vi "MLP_FS_ Target.vi"   [LabVIEW 2022 SP3]
uses:
  <vilib>/rvi/Emulation/niFpgaEmulationIsFPGAContextNoSignature.vi
  <vilib>/rvi/DataTransferAndStorage/Container/Common/niFpgaContainerGetUniqueNameForEmu.vi
  <vilib>/rvi/Memory/Memory_Emulation/niFpgaMemoryEmulationCacheClearOnFirstRun.vi
  <vilib>/rvi/Memory/Memory_Emulation/nirvimemoryEmulationManagerCache_MakeExclusive.vi
  <vilib>/rvi/Memory/Memory_Emulation/niFpgaMemoryEmulationValidateCache.vi
  <vilib>/rvi/Memory/Memory_Emulation/nirvimemoryEmulationManagerCache_InsertValue.vi
  <vilib>/Utility/error.llb/Clear Errors.vi
  <vilib>/rvi/Memory/Memory_Emulation/nirvimemoryEmulationManagerCache_ReleaseExclusive.vi
  <vilib>/rvi/Memory/Memory_Emulation/nirvimemoryEmulationManagerCache_GetValue.vi
  <vilib>/rvi/Memory/Memory_Emulation/nirvimemoryEmulationManagerCache_SetValue.vi
  <vilib>/rvi/Emulation/niFpgaProcessEmulError.vi
  <vilib>/rvi/Emulation/niFpgaSctlEmulationGetInTimedLoop.vi
  <vilib>/rvi/interface/RandomDataEmulation/niFpgaRandomDataHandleErrors.vi
  <vilib>/rvi/Memory/Memory_Emulation/nirvimemoryFastEmulation.vi
  <vilib>/rvi/Memory/Memory_Emulation/nirvimemoryEmulation.vi
  <vilib>/rvi/errors/nirviReportUnexpectedCaseInternalError (U32).vi
  <vilib>/rvi/DataTransferAndStorage/Container/XNode/niFpgaContainer.xnode
  <vilib>/rvi/DataTransferAndStorage/Register/Emulation/niFpgaRegisterEmulation.vi
  <vilib>/rvi/interface/RandomDataEmulation/nirviRandomDataFpgaReadWriteTemplate.vi
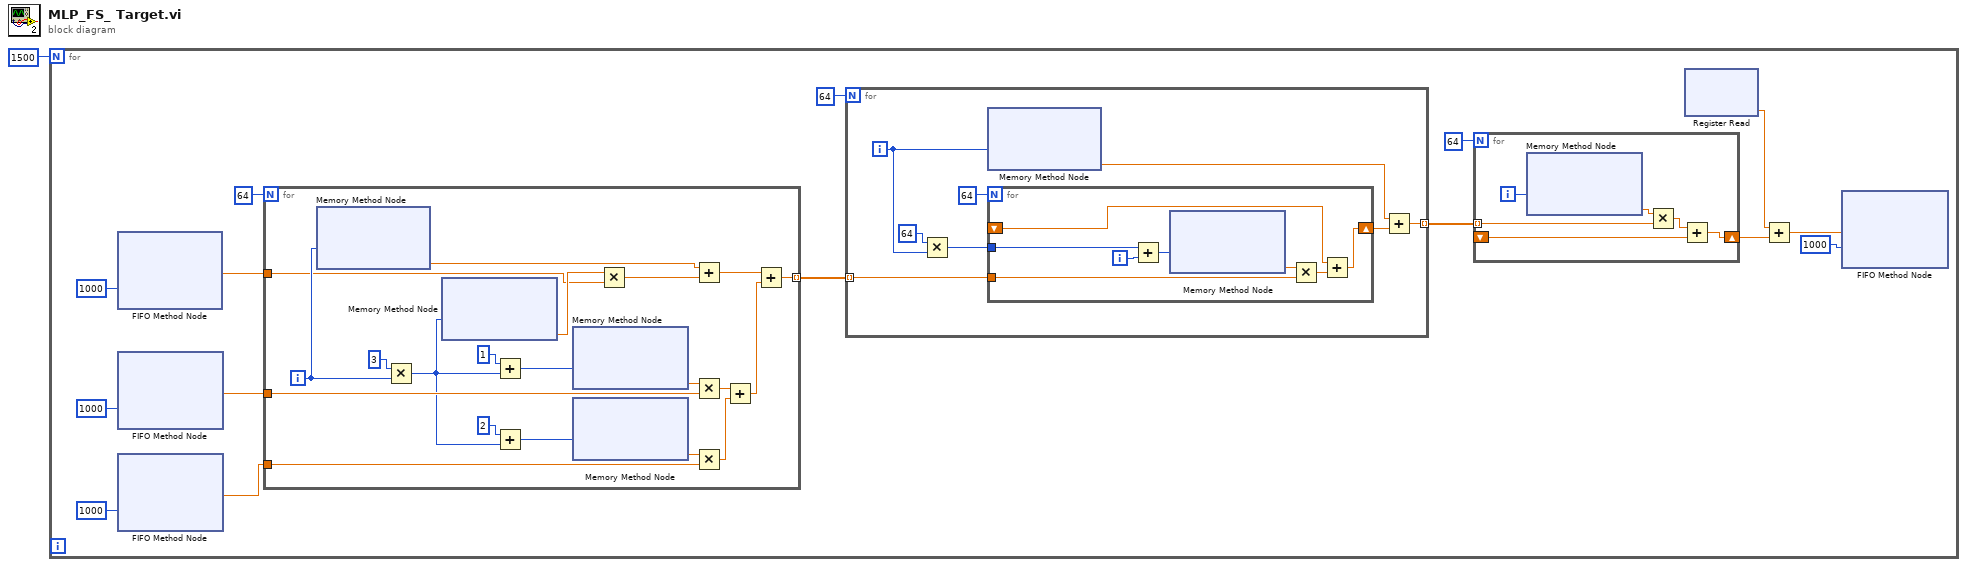
[diagram p0: block diagram]
diagram:
  n1 = for {
    N: 1500 -> [_]
    n2 = xnode ("FIFO Method Node")("Timeout"=1000) -> ("Element"=w2:sgl)  [unwired: 1 in, 2 out]
    n3 = xnode ("FIFO Method Node")("Timeout"=1000) -> ("Element"=w13:sgl)  [unwired: 1 in, 2 out]
    n4 = xnode ("FIFO Method Node")("Timeout"=1000) -> ("Element"=w12:sgl)  [unwired: 1 in, 2 out]
    n5 = for {
      N: 64 -> [_]
      tunnel: w13 -> [w58]
      tunnel: w12 -> [w57]
      tunnel: [w51] -> w10 mode=indexing
      tunnel: w2 -> [w39]
      i -> [w46]
      n6 = xnode ("Memory Method Node")("Address"=w46) -> ("Data"=w50:sgl)  [unwired: 1 in, 1 out]
      n7 = Multiply(x=3, y=w46) -> (x*y=w44:i32)
      n8 = xnode ("Memory Method Node")("Address"=w44) -> ("Data"=w49:sgl)  [unwired: 1 in, 1 out]
      n9 = Add(x=1, y=w44) -> (x+y=w40:i32)
      n10 = Add(x=2, y=w44) -> (x+y=w41:i32)
      n11 = xnode ("Memory Method Node")("Address"=w40) -> ("Data"=w48:sgl)  [unwired: 1 in, 1 out]
      n12 = xnode ("Memory Method Node")("Address"=w41) -> ("Data"=w47:sgl)  [unwired: 1 in, 1 out]
      n13 = Multiply(x=w49, y=w39) -> (x*y=w54:sgl)
      n14 = Add(x=w50, y=w54) -> (x+y=w53:sgl)
      n15 = Multiply(x=w48, y=w58) -> (x*y=w55:sgl)
      n16 = Multiply(x=w47, y=w57) -> (x*y=w56:sgl)
      n17 = Add(x=w55, y=w56) -> (x+y=w52:sgl)
      n18 = Add(x=w53, y=w52) -> (x+y=w51:sgl)
    }
    n19 = for {
      N: 64 -> [_]
      tunnel: w10 -> [w27] mode=indexing
      tunnel: [w30] -> w8 mode=indexing
      i -> [w25]
      n20 = Multiply(x=64, y=w25) -> (x*y=w26:i32)
      n21 = xnode ("Memory Method Node")("Address"=w25) -> ("Data"=w29:sgl)  [unwired: 1 in, 1 out]
      n22 = for {
        N: 64 -> [_]
        tunnel: w27 -> [w38]
        tunnel: w26 -> [w34]
        shift-right: [w32] -> w23
        shift-left: _ -> [w31]
        i -> [w36]
        n23 = Add(x=w34, y=w36) -> (x+y=w35:i32)
        n24 = xnode ("Memory Method Node")("Address"=w35) -> ("Data"=w37:sgl)  [unwired: 1 in, 1 out]
        n25 = Multiply(x=w37, y=w38) -> (x*y=w33:sgl)
        n26 = Add(x=w31, y=w33) -> (x+y=w32:sgl)
      }
      n27 = Add(x=w29, y=w23) -> (x+y=w30:sgl)
    }
    n28 = for {
      N: 64 -> [_]
      tunnel: w8 -> [w22] mode=indexing
      shift-right: [w19] -> w7
      shift-left: _ -> [w20]
      i -> [w17]
      n29 = xnode ("Memory Method Node")("Address"=w17) -> ("Data"=w18:sgl)  [unwired: 1 in, 1 out]
      n30 = Multiply(x=w18, y=w22) -> (x*y=w21:sgl)
      n31 = Add(x=w21, y=w20) -> (x+y=w19:sgl)
    }
    n32 = xnode ("Register Read")() -> ("Data"=w5:sgl)  [unwired: 1 in, 1 out]
    n33 = Add(x=w5, y=w7) -> (x+y=w6:sgl)
    n34 = xnode ("FIFO Method Node")("Element"=w6, "Timeout"=1000) -> ()  [unwired: 1 in, 2 out]
  }
